vi "AUTON_Index.vi"(0 "Auton Array":dbl[][](array[numeric]), 5 "MeasuredHeading":dbl, 7 "LeftEncoder":dbl, 9 "RightEncoder":dbl) -> (4 "Right Drive":dbl, 6 "Left Drive":dbl, 8 "Harvester":dbl, 10 "Winch":dbl, 14 "Roller":dbl, 15 "Cam":dbl)   [LabVIEW 2013]
uses:
  Robot Global Data.vi
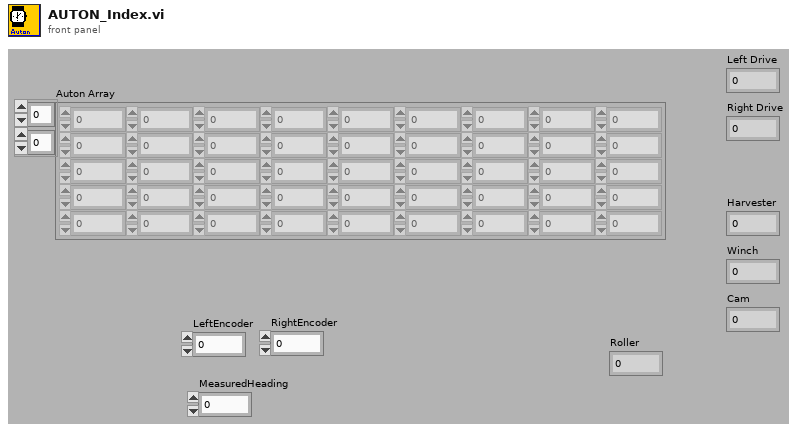
[diagram p1: front panel]
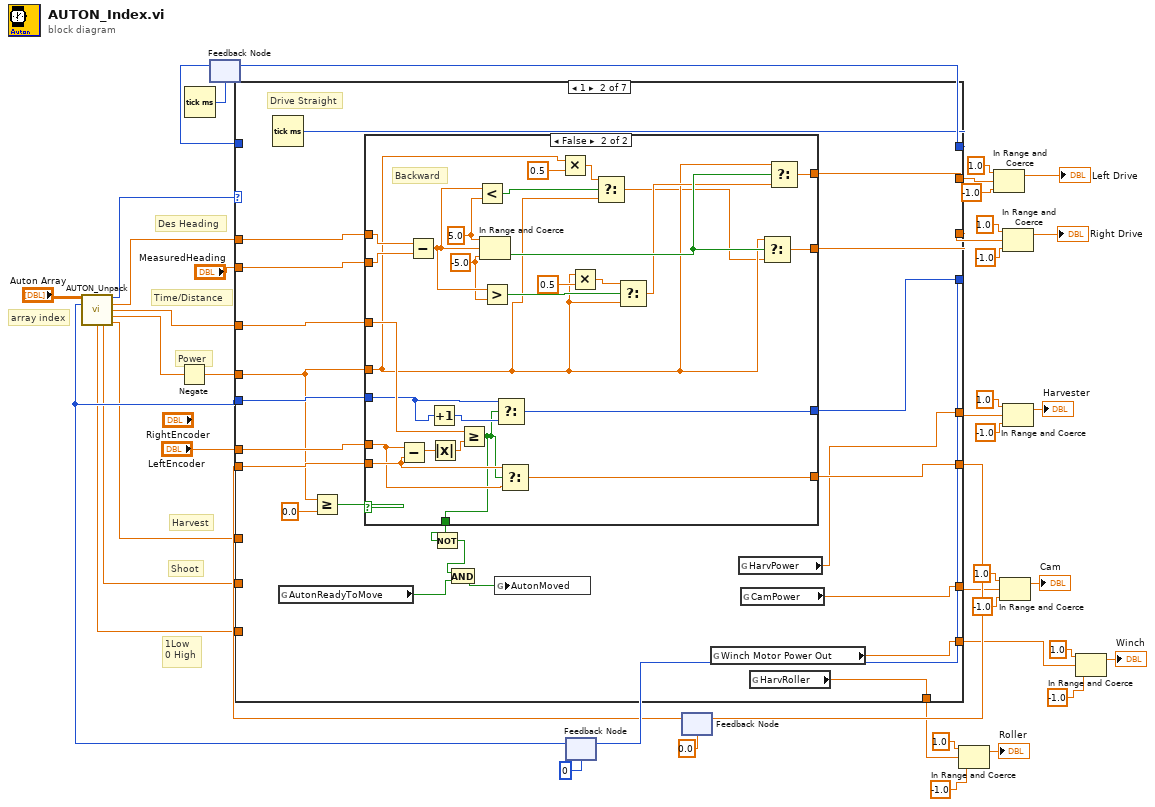
[diagram p0: block diagram]
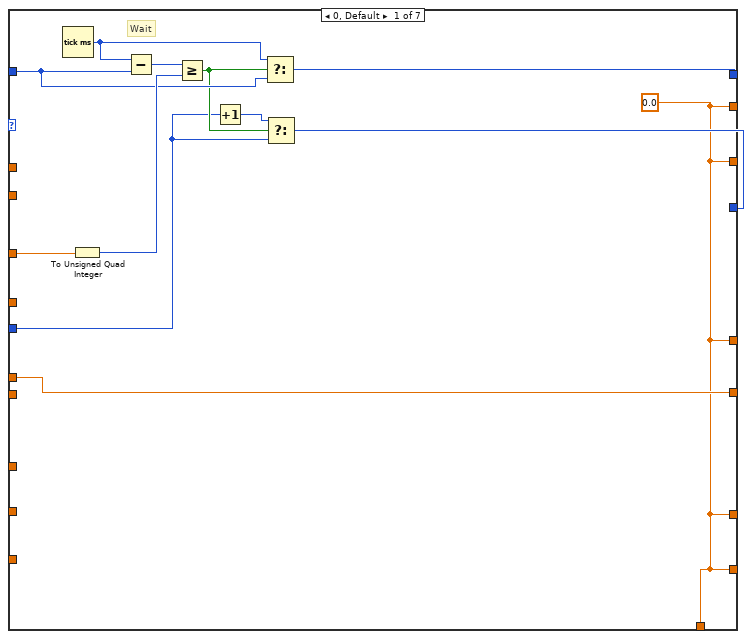
[diagram p2: hidden frame]
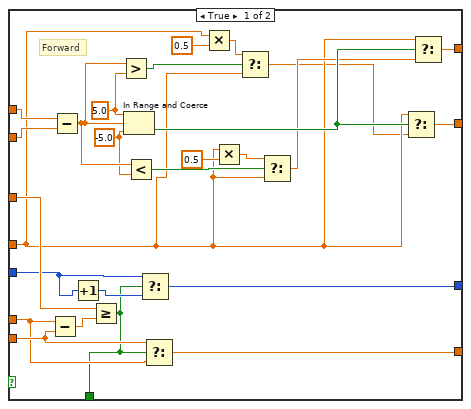
[diagram p3: hidden frame]
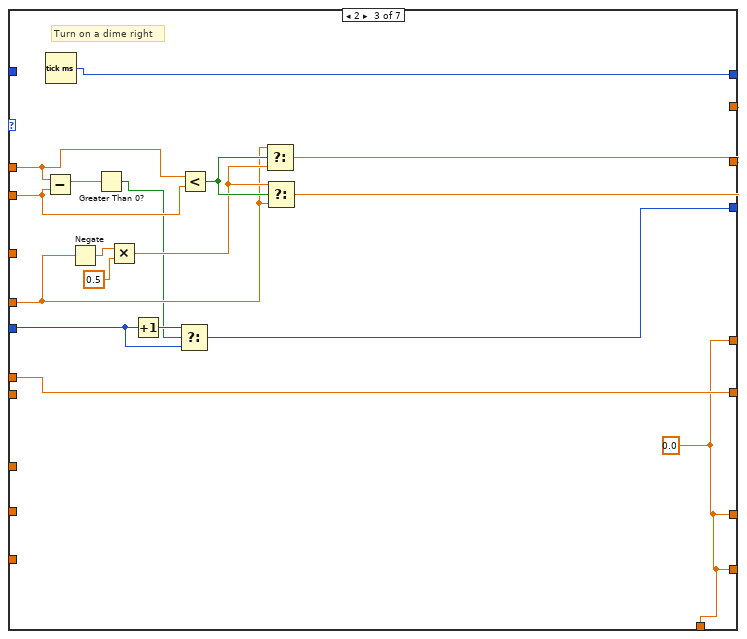
[diagram p4: hidden frame]
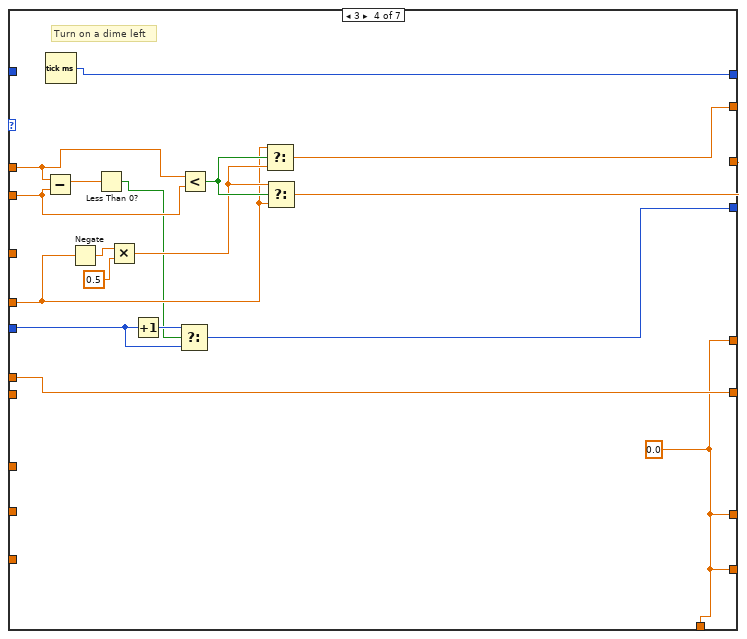
[diagram p5: hidden frame]
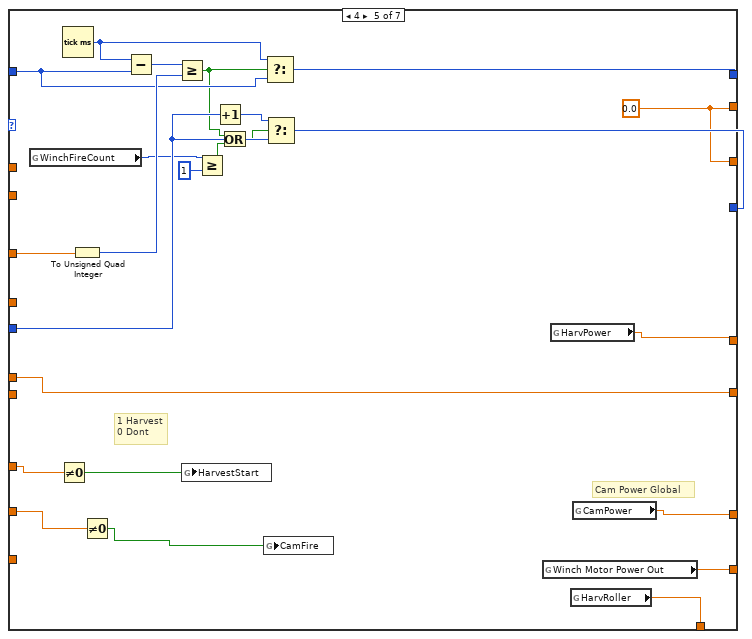
[diagram p6: hidden frame]
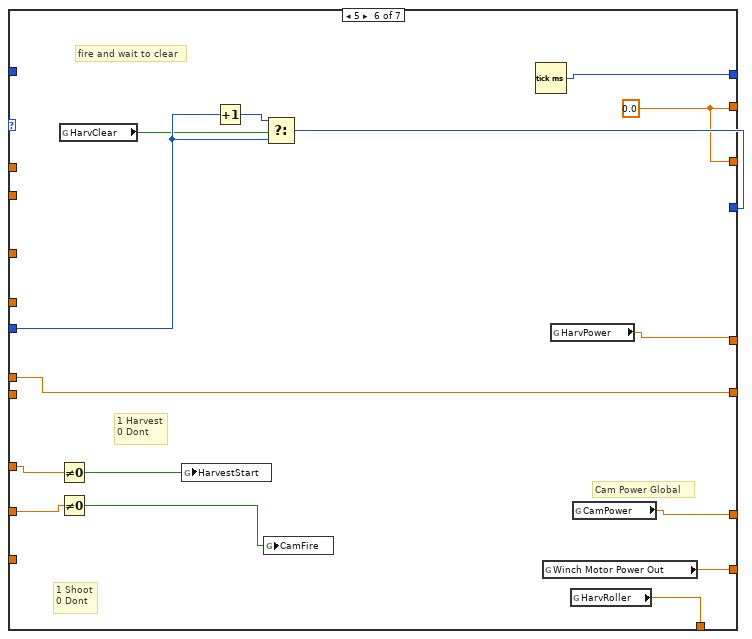
[diagram p7: hidden frame]
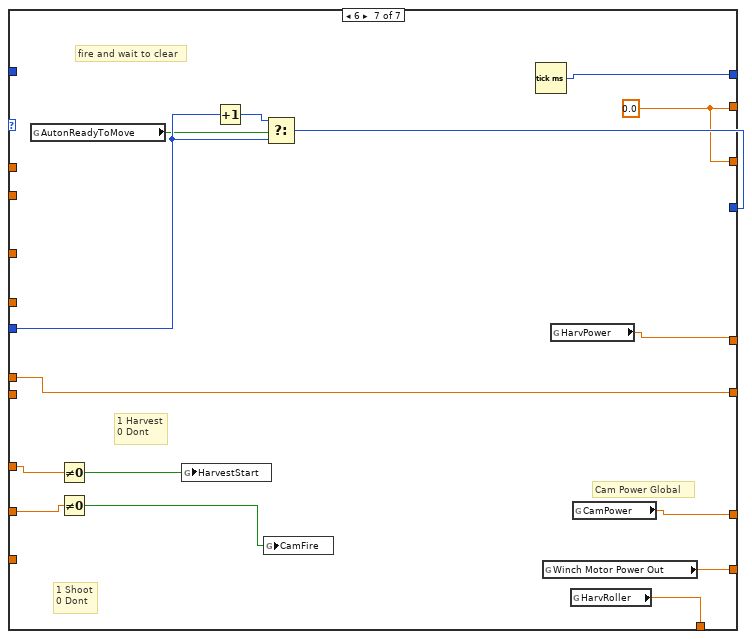
[diagram p8: hidden frame]
diagram:
  # "1Low\n0 High"
  # "Shoot"
  # "Harvest"
  # "Des Heading"
  # "Time/Distance"
  # "Power"
  # "array index"
  n1 = Tick Count (ms)() -> (millisecond timer value=w42:u32)
  n2 = feedback #1(w42) -> (w43:u32)
  n3 = feedback #2(0) -> (w23:i32)
  n4 = call "AUTON_Unpack.vi"("all rows"="Auton Array", "Index"=w23) -> ("Primitive ID"=w26:i16, "Desired Heading"=w25:dbl, "Time/Distance"=w24:dbl, "Power"=w11:dbl, "LowGear"=w1:dbl, "Shoot"=w8:dbl, "Harvest"=w9:dbl)  [unwired: 7 in]
  n5 = Negate(x=w11) -> (-x=w10:dbl)
  n6 = feedback #3(0.0) -> (w28:dbl)
  n7 = case shown="1" w26 {
    tunnel: [w48 w76 w143 w160 w182 w202 w217] -> w30
    tunnel: w23 -> [w49 w71 w146 w163 w183 w203 w218]
    tunnel: [w56 w68 w148 w165 w189 w193 w208] -> w32
    tunnel: w43 -> [w53 _ _ _ w186 _ _]
    tunnel: w24 -> [w47 w77 _ _ w181 _ _]
    tunnel: w25 -> [_ w75 w141 w158 _ _ _]
    tunnel: [w45 w73 w144 w161 w180 w201 w216] -> w40
    tunnel: [w45 w72 w145 w162 w180 w201 w216] -> w33
    tunnel: w10 -> [_ w67 w135 w152 _ _ _]
    tunnel: "LeftEncoder" -> [w46 w69 w142 w159 w179 w200 w215]
    tunnel: "MeasuredHeading" -> [_ w74 w140 w157 _ _ _]
    tunnel: w28 -> [_ w70 _ _ _ _ _]
    tunnel: [w46 w78 w142 w159 w179 w200 w215] -> w27
    tunnel: [w45 w64 w132 w149 w177 w198 w213] -> w13
    tunnel: [w45 w62 w132 w149 w178 w199 w214] -> w12
    tunnel: w9 -> [_ _ _ _ w174 w196 w211]
    tunnel: w8 -> [_ _ _ _ w176 w191 w206]
    tunnel: [w45 w63 w132 w149 w175 w197 w212] -> w7
    tunnel: [w45 w61 w132 w149 w171 w194 w209] -> w3
    tunnel: w1 -> [_ _ _ _ _ _ _]
    frame 0, Default {
      w45 = 0.0 ("Numeric")
      # "Wait"
      n8 = Tick Count (ms)() -> (millisecond timer value=w52:u32)
      n9 = To Unsigned Quad Integer(1:w47) -> (0:w54:u64)
      n10 = Subtract(x=w52, y=w53) -> (x-y=w55:u32)
      n11 = Greater Or Equal?(x=w55, y=w54) -> (x >= y?=w51:bool)
      n12 = Increment(x=w49) -> (x+1=w50:i32)
      n13 = Select(t=w52, s=w51, f=w53) -> (s? t:f=w56:u32)
      n14 = Select(t=w50, s=w51, f=w49) -> (s? t:f=w48:i32)
    }
    frame 1 {
      # "Drive Straight"
      n15 = Tick Count (ms)() -> (millisecond timer value=w68:u32)
      n16 = global read "Robot Global Data.vi" "AutonReadyToMove"() -> (w60:bool)
      n17 = Greater Or Equal?(x=w67, y=0.0) -> (x >= y?=w65:bool)
      n18 = case shown="False" w65 {
        tunnel: [w104 w131] -> w78
        tunnel: w77 -> [w102 w130]
        tunnel: [w101 w129] -> w76
        tunnel: w75 -> [w100 w128]
        tunnel: w74 -> [w99 w127]
        tunnel: [w97 w125] -> w73
        tunnel: [w96 w124] -> w72
        tunnel: w67 -> [w85 w113]
        tunnel: w71 -> [w82 w110]
        tunnel: w70 -> [w81 w109]
        tunnel: w69 -> [w80 w108]
        tunnel: [w79 w105] -> w57
        frame True {
          w93 = -5.0 ("lower limit")
          w95 = 5.0 ("upper limit")
          # "Forward"
          n19 = Subtract(x=w80, y=w81) -> (x-y=w103:dbl)
          n20 = Subtract(x=w100, y=w99) -> (x-y=w94:dbl)
          n21 = Increment(x=w82) -> (x+1=w83:i32)
          n22 = Greater Or Equal?(x=w102, y=w103) -> (x >= y?=w79:bool)
          n23 = Greater?(x=w94, y=w95) -> (0:w88:bool)
          n24 = In Range and Coerce(upper limit=w95, x=w94, lower limit=w93) -> (In Range?=w98:bool)  [unwired: 1 out]
          n25 = Less?(x=w94, y=w93) -> (x < y?=w92:bool)
          n26 = Select(t=w82, s=w79, f=w83) -> (s? t:f=w101:i32)
          n27 = Select(t=w81, s=w79, f=w80) -> (s? t:f=w104:dbl)
          n28 = Multiply(x=w85, y=0.5) -> (x*y=w87:dbl)
          n29 = Multiply(x=w85, y=0.5) -> (x*y=w90:dbl)
          n30 = Select(t=w87, s=w88, f=w85) -> (s? t:f=w84:dbl)
          n31 = Select(t=w90, s=w92, f=w85) -> (s? t:f=w89:dbl)
          n32 = Select(t=w85, s=w98, f=w84) -> (s? t:f=w96:dbl)
          n33 = Select(t=w85, s=w98, f=w89) -> (s? t:f=w97:dbl)
        }
        frame False {
          w121 = -5.0 ("lower limit")
          w123 = 5.0 ("upper limit")
          # "Backward"
          n34 = Subtract(x=w108, y=w109) -> (x-y=w106:dbl)
          n35 = Subtract(x=w128, y=w127) -> (x-y=w122:dbl)
          n36 = Increment(x=w110) -> (x+1=w111:i32)
          n37 = Absolute Value(x=w106) -> (abs(x)=w107:dbl)
          n38 = Greater Or Equal?(x=w130, y=w107) -> (x >= y?=w105:bool)
          n39 = Less?(x=w122, y=w123) -> (x < y?=w116:bool)
          n40 = In Range and Coerce(upper limit=w123, x=w122, lower limit=w121) -> (In Range?=w126:bool)  [unwired: 1 out]
          n41 = Greater?(x=w122, y=w121) -> (0:w120:bool)
          n42 = Select(t=w110, s=w105, f=w111) -> (s? t:f=w129:i32)
          n43 = Select(t=w109, s=w105, f=w108) -> (s? t:f=w131:dbl)
          n44 = Multiply(x=w113, y=0.5) -> (x*y=w115:dbl)
          n45 = Multiply(x=w113, y=0.5) -> (x*y=w118:dbl)
          n46 = Select(t=w115, s=w116, f=w113) -> (s? t:f=w112:dbl)
          n47 = Select(t=w118, s=w120, f=w113) -> (s? t:f=w117:dbl)
          n48 = Select(t=w113, s=w126, f=w112) -> (s? t:f=w124:dbl)
          n49 = Select(t=w113, s=w126, f=w117) -> (s? t:f=w125:dbl)
        }
      }
      n50 = Not(x=w57) -> (.not. x?=w58:bool)
      n51 = And(x=w58, y=w60) -> (x .and. y?=w59:bool)
      n52 = global write "Robot Global Data.vi" "AutonMoved"(w59) -> ()
      n53 = global read "Robot Global Data.vi" "Winch Motor Power Out"() -> (w63:dbl)
      n54 = global read "Robot Global Data.vi" "HarvPower"() -> (w62:dbl)
      n55 = global read "Robot Global Data.vi" "CamPower"() -> (w64:dbl)
      n56 = global read "Robot Global Data.vi" "HarvRoller"() -> (w61:dbl)
    }
    frame 2 {
      w132 = 0.0 ("Numeric")
      # "Turn on a dime right"
      n57 = Subtract(x=w141, y=w140) -> (x-y=w134:dbl)
      n58 = Tick Count (ms)() -> (millisecond timer value=w148:u32)
      n59 = Negate(x=w135) -> (-x=w138:dbl)
      n60 = Greater Than 0?(x=w134) -> (x > 0?=w133:bool)
      n61 = Multiply(x=w138, y=0.5) -> (x*y=w136:dbl)
      n62 = Increment(x=w146) -> (x+1=w147:i32)
      n63 = Select(t=w147, s=w133, f=w146) -> (s? t:f=w143:i32)
      n64 = Less?(x=w141, y=w140) -> (x < y?=w139:bool)
      n65 = Select(t=w135, s=w139, f=w136) -> (s? t:f=w144:dbl)
      n66 = Select(t=w136, s=w139, f=w135) -> (s? t:f=w145:dbl)
    }
    frame 3 {
      w149 = 0.0 ("Numeric")
      # "Turn on a dime left"
      n67 = Subtract(x=w158, y=w157) -> (x-y=w151:dbl)
      n68 = Tick Count (ms)() -> (millisecond timer value=w165:u32)
      n69 = Negate(x=w152) -> (-x=w155:dbl)
      n70 = Less Than 0?(x=w151) -> (x < 0?=w150:bool)
      n71 = Multiply(x=w155, y=0.5) -> (x*y=w153:dbl)
      n72 = Increment(x=w163) -> (x+1=w164:i32)
      n73 = Select(t=w164, s=w150, f=w163) -> (s? t:f=w160:i32)
      n74 = Less?(x=w158, y=w157) -> (x < y?=w156:bool)
      n75 = Select(t=w152, s=w156, f=w153) -> (s? t:f=w161:dbl)
      n76 = Select(t=w153, s=w156, f=w152) -> (s? t:f=w162:dbl)
    }
    frame 4 {
      w180 = 0.0 ("Numeric")
      # "1 Harvest\n0 Dont"
      # "Cam Power Global"
      n77 = global read "Robot Global Data.vi" "WinchFireCount"() -> (w167:i32)
      n78 = Not Equal To 0?(x=w174) -> (x != 0?=w173:bool)
      n79 = Tick Count (ms)() -> (millisecond timer value=w185:u32)
      n80 = To Unsigned Quad Integer(1:w181) -> (0:w187:u64)
      n81 = Not Equal To 0?(x=w176) -> (x != 0?=w172:bool)
      n82 = Subtract(x=w185, y=w186) -> (x-y=w188:u32)
      n83 = Greater Or Equal?(x=w188, y=w187) -> (x >= y?=w169:bool)
      n84 = global write "Robot Global Data.vi" "HarvestStart"(w173) -> ()
      n85 = Greater Or Equal?(x=w167, y=1) -> (x >= y?=w168:bool)
      n86 = Increment(x=w183) -> (x+1=w184:i32)
      n87 = Or(x=w169, y=w168) -> (x .or. y?=w170:bool)
      n88 = global write "Robot Global Data.vi" "CamFire"(w172) -> ()
      n89 = Select(t=w185, s=w169, f=w186) -> (s? t:f=w189:u32)
      n90 = Select(t=w184, s=w170, f=w183) -> (s? t:f=w182:i32)
      n91 = global read "Robot Global Data.vi" "Winch Motor Power Out"() -> (w175:dbl)
      n92 = global read "Robot Global Data.vi" "HarvPower"() -> (w178:dbl)
      n93 = global read "Robot Global Data.vi" "HarvRoller"() -> (w171:dbl)
      n94 = global read "Robot Global Data.vi" "CamPower"() -> (w177:dbl)
    }
    frame 5 {
      w201 = 0.0 ("Numeric")
      # "fire and wait to clear"
      # "1 Harvest\n0 Dont"
      # "1 Shoot\n0 Dont"
      # "Cam Power Global"
      n95 = Not Equal To 0?(x=w196) -> (x != 0?=w195:bool)
      n96 = Not Equal To 0?(x=w191) -> (x != 0?=w190:bool)
      n97 = global read "Robot Global Data.vi" "HarvClear"() -> (w192:bool)
      n98 = global write "Robot Global Data.vi" "HarvestStart"(w195) -> ()
      n99 = Increment(x=w203) -> (x+1=w204:i32)
      n100 = global write "Robot Global Data.vi" "CamFire"(w190) -> ()
      n101 = Select(t=w204, s=w192, f=w203) -> (s? t:f=w202:i32)
      n102 = Tick Count (ms)() -> (millisecond timer value=w193:u32)
      n103 = global read "Robot Global Data.vi" "Winch Motor Power Out"() -> (w197:dbl)
      n104 = global read "Robot Global Data.vi" "HarvPower"() -> (w199:dbl)
      n105 = global read "Robot Global Data.vi" "HarvRoller"() -> (w194:dbl)
      n106 = global read "Robot Global Data.vi" "CamPower"() -> (w198:dbl)
    }
    frame 6 {
      w216 = 0.0 ("Numeric")
      # "fire and wait to clear"
      # "1 Harvest\n0 Dont"
      # "1 Shoot\n0 Dont"
      # "Cam Power Global"
      n107 = global read "Robot Global Data.vi" "AutonReadyToMove"() -> (w207:bool)
      n108 = Not Equal To 0?(x=w211) -> (x != 0?=w210:bool)
      n109 = Not Equal To 0?(x=w206) -> (x != 0?=w205:bool)
      n110 = global write "Robot Global Data.vi" "HarvestStart"(w210) -> ()
      n111 = Increment(x=w218) -> (x+1=w219:i32)
      n112 = global write "Robot Global Data.vi" "CamFire"(w205) -> ()
      n113 = Select(t=w219, s=w207, f=w218) -> (s? t:f=w217:i32)
      n114 = Tick Count (ms)() -> (millisecond timer value=w208:u32)
      n115 = global read "Robot Global Data.vi" "Winch Motor Power Out"() -> (w212:dbl)
      n116 = global read "Robot Global Data.vi" "HarvPower"() -> (w214:dbl)
      n117 = global read "Robot Global Data.vi" "HarvRoller"() -> (w209:dbl)
      n118 = global read "Robot Global Data.vi" "CamPower"() -> (w213:dbl)
    }
  }
  n119 = feedback-in #1(w32) -> ()
  n120 = feedback-in #2(w30) -> ()
  n121 = feedback-in #3(w27) -> ()
  n122 = In Range and Coerce(upper limit=1.0, x=w3, lower limit=-1.0) -> (coerced(x)=→"Roller":dbl)  [unwired: 1 out]
  n123 = In Range and Coerce(upper limit=1.0, x=w40, lower limit=-1.0) -> (coerced(x)=→"Left Drive":dbl)  [unwired: 1 out]
  n124 = In Range and Coerce(upper limit=1.0, x=w13, lower limit=-1.0) -> (coerced(x)=→"Cam":dbl)  [unwired: 1 out]
  n125 = In Range and Coerce(upper limit=1.0, x=w33, lower limit=-1.0) -> (coerced(x)=→"Right Drive":dbl)  [unwired: 1 out]
  n126 = In Range and Coerce(upper limit=1.0, x=w12, lower limit=-1.0) -> (coerced(x)=→"Harvester":dbl)  [unwired: 1 out]
  n127 = In Range and Coerce(upper limit=1.0, x=w7, lower limit=-1.0) -> (coerced(x)=→"Winch":dbl)  [unwired: 1 out]
